vi "Utility_Calculate_PS.vi"(5 "input_2":dbl=84000.0, 7 "input_1":dbl=6.772222028271756, 8 "error in":errorcluster, 9 "units":enum16{"SI", "IP"}(ring), 10 "InpCode":T3(ring)=enum."PS", 11 "Mixure Cluster":T1={"Mixture Name"="Air (dry)", "Molecular weight (g/mol)"=28.958600656, "Critical temperature (K)"=132.83069752889762, "Critical Pressure (kPa)"=3852.042257237323, "Critical Density (mol/L)"=0.0, "# Components"=3, "Fluid File Paths"=[path "C:/Users/ASITest/Desktop/REFPROP/fluids/NITROGEN.FLD", path "C:/Users/ASITest/Desktop/REFPROP/fluids/ARGON.FLD", path "C:/Users/ASITest/Desktop/REFPROP/fluids/OXYGEN.FLD"], "Component molar fractions"=[0.7812, 0.0092, 0.2096], "Refprop Main Directory"=path "C:/Users/ASITest/Desktop/REFPROP", "DLL Version Number"=10.0}) -> (0 "error out":errorcluster={"status"=TRUE, "code"=17, "source"="REFPROP_ErrorConverter.vi<ERR>\nOne or more inputs are out of range; Temperature above 1.5x(upper limit): T = 10181.4 K, Tmax = 1993.69 K.                                                                                                                                                    \n\n\n<b>Complete call chain:</b>\r\n     REFPROP_ErrorConverter.vi\r\n     PSFLSHdll.vi\r\n     Utility_Calculate_PS.vi"}, 2 "INFO_OUT":T2={"icomp out"=3, "wmm out"=0.0, "ttrp out"=0.0, "tnbpt out"=0.0, "tc out"=0.0, "pc out"=0.0, "dc out"=0.0, "Zc out"=0.0, "acf out"=0.0, "dip out"=0.0, "Rgas out"=0.0}, 3 "dataout":dbl[](array[numeric])=[9908.201736464158, 6.772222028271756, 13169.831204666785, 84000.0, 0.0023166880524800003, 0.0023166880524800003, 10246.596882712158, 1.0691855582717507, 1.3563012835972652, 1925.6787564705157, 998.0])   [LabVIEW 2016]
doc: "Utility function that provides access to all of the functionality contained in the FLSH and SAT polymorphic VIs. \n\nPlease feel free to contact me if you have any questions .\nMy mail:ken_pop@tom.com yan.ding@jci.com"
uses:
  Ctl/Mixture Composition cluster_d.ctl
  Ctl/variable_refprop.ctl
  Ctl/FLSH_Inputs.ctl
  VIs/PSFLSHdll.vi
  VIs/HSFLSHdll.vi
  VIs/SATTdll.vi
  VIs/SATPdll.vi
  VIs/TPFLSHdll.vi
  VIs/THFLSHdll.vi
  VIs/TSFLSHdll.vi
  VIs/PHFLSHdll.vi
  VIs/PQFLSHdll.vi
  VIs/TQFLSHdll.vi
panel:
  out "n":i32=3
  out "wm":dbl=28.958600656
  out "x":dbl[](array[numeric])=[0.7812, 0.0092, 0.2096]
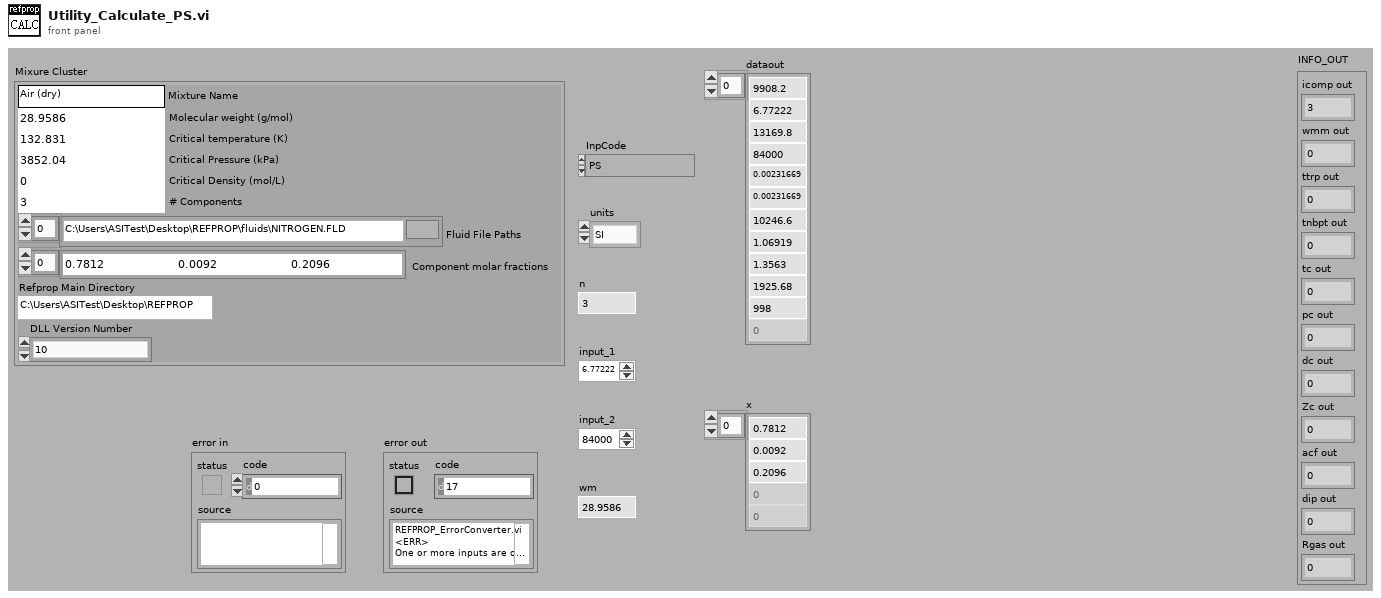
[diagram p1: front panel]
types:
  T1 = typedef "Mixture Composition cluster_d.ctl" = cluster{"Mixture Name":string, "Molecular weight (g/mol)":dbl, "Critical temperature (K)":dbl, "Critical Pressure (kPa)":dbl, "Critical Density (mol/L)":dbl, "# Components":i32, "Fluid File Paths":path[], "Component molar fractions":dbl[], "Refprop Main Directory":path, "DLL Version Number":dbl}
  T2 = cluster{"icomp out":i32, "wmm out":dbl, "ttrp out":dbl, "tnbpt out":dbl, "tc out":dbl, "pc out":dbl, "dc out":dbl, "Zc out":dbl, "acf out":dbl, "dip out":dbl, "Rgas out":dbl}
  T3 = enum16{"0", "PS", "HS", "T", "P", "TP", "TH", "TS", "PH", "PQ", "TQ"}
  T4 = typedef "FLSH_Inputs.ctl" = cluster{"t":dbl, "p":dbl, "e":dbl, "h":dbl, "s":dbl, "q":dbl, "z":dbl[], "kq":i32, "kr":i32, "D":dbl}
  T5 = typedef "variable_refprop.ctl" = cluster{"t":dbl, "p":dbl, "z":dbl[], "d":dbl, "D":dbl, "Dl":dbl, "Dv":dbl, "x":dbl[], "y":dbl[], "q":dbl, "e":dbl, "h":dbl, "s":dbl, "Cv":dbl, "Cp":dbl, "w":dbl, "ierr":i32, "herr":string, "i":i32, "z":dbl, "kq":i32, "kph":i32, "kr":i32, "nroot":i32, "k1":i32, "t1":dbl, "p1":dbl, "d1":dbl, "k2":i32, "t2":dbl, "p2":dbl, "d2":dbl, "k3":i32, "t3":dbl, "p3":dbl, "d3":dbl, "iGuess":dbl}
  T6 = typedef "FLSH_Outputs.ctl" = cluster{"t":dbl, "p":dbl, "D":dbl, "Dl":dbl, "Dv":dbl, "x":dbl[], "y":dbl[], "q":dbl, "e":dbl, "h":dbl, "s":dbl, "Cv":dbl, "Cp":dbl, "w":dbl, "ierr":i32, "herr":string, "herr_Length":i32}
  T7 = typedef "SAT_Outputs.ctl" = cluster{"D":dbl, "e":dbl, "h":dbl, "p":dbl, "s":dbl, "t":dbl, "q":dbl, "Dl":dbl, "Dv":dbl, "x":dbl[], "y":dbl[], "nroot":i32, "k1":i32, "t1":dbl, "p1":dbl, "d1":dbl, "k2":i32, "t2":dbl, "p2":dbl, "d2":dbl, "k3":i32, "t3":dbl, "p3":dbl, "d3":dbl, "ierr":i32, "herr":string, "herr_length":i32}
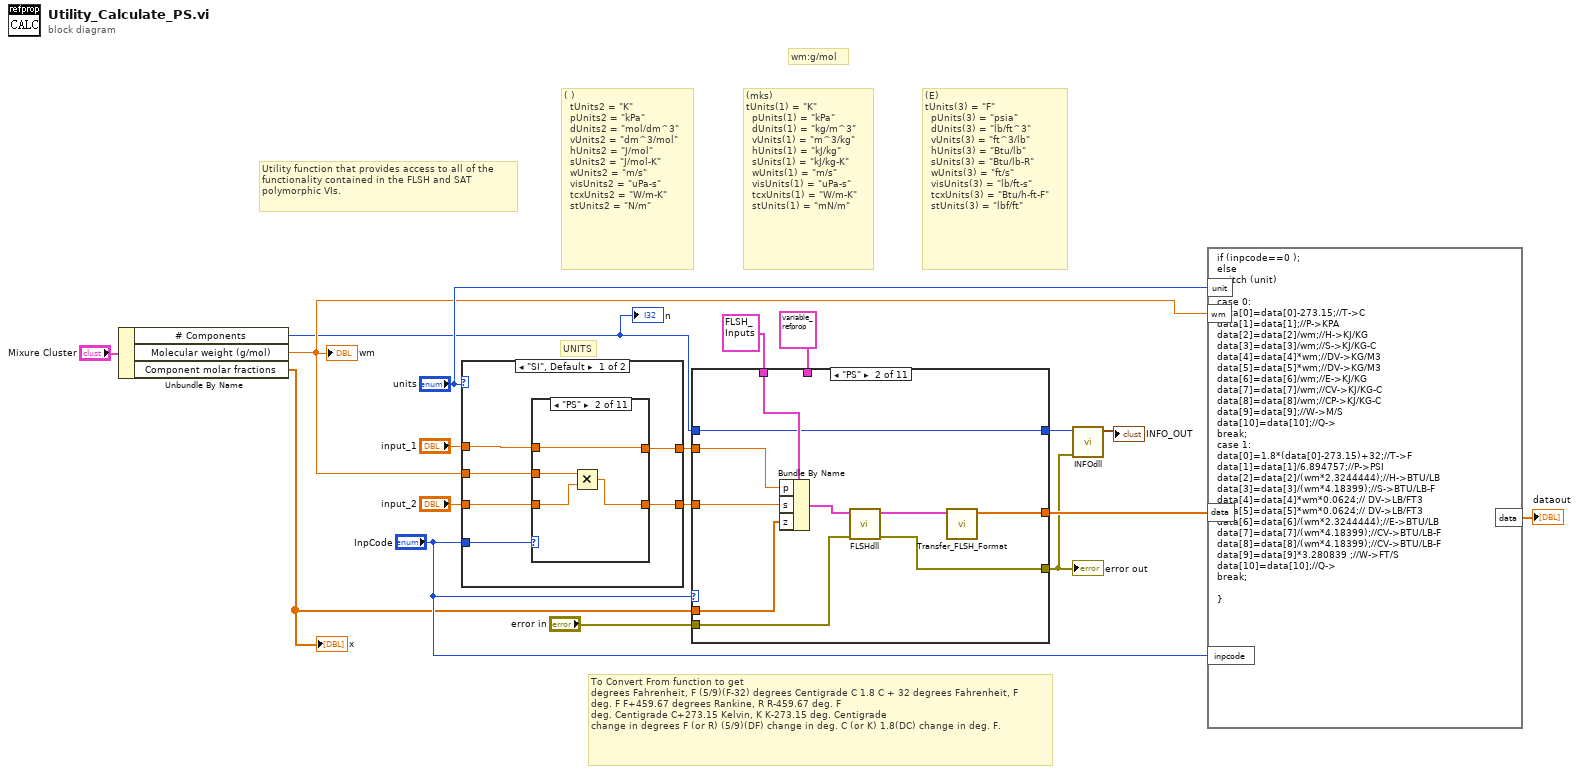
[diagram p0: block diagram]
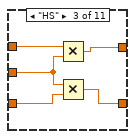
[diagram p3: hidden frame]
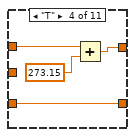
[diagram p4: hidden frame]
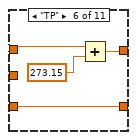
[diagram p6: hidden frame]
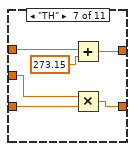
[diagram p7: hidden frame]
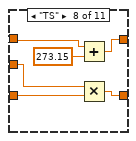
[diagram p8: hidden frame]
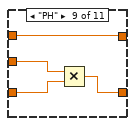
[diagram p9: hidden frame]
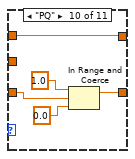
[diagram p10: hidden frame]
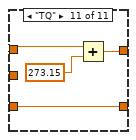
[diagram p11: hidden frame]
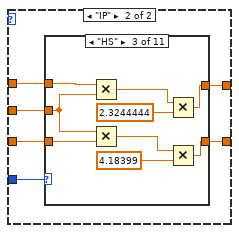
[diagram p12: hidden frame]
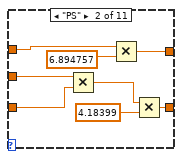
[diagram p14: hidden frame]
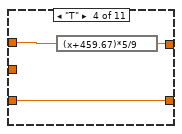
[diagram p15: hidden frame]
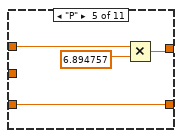
[diagram p16: hidden frame]
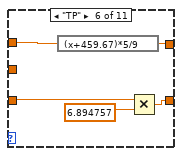
[diagram p17: hidden frame]
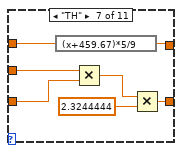
[diagram p18: hidden frame]
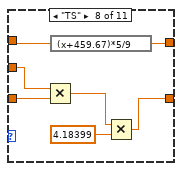
[diagram p19: hidden frame]
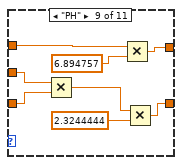
[diagram p20: hidden frame]
diagram:
  # "Utility function that provides access to all of the functionality contained in the FLSH and SAT polymorphic VIs."
  # "To Convert From function to get \ndegrees Fahrenheit, F (5/9)(F-32) degrees Centigrade C 1.8 C + 32 degrees Fahrenheit, F \ndeg. F F+459.67 degrees Rankine, R R-459.67 deg. F \ndeg. Centigrade C+273.15 Kelvin, K K-273.15 deg. Centigrade \nchange in degrees F (or R) (5/9)(DF) change in deg. C (or K) 1.8(DC) change in deg. F."
  # "(E)\ntUnits(3) = \"F\"\n  pUnits(3) = \"psia\"\n  dUnits(3) = \"lb/ft^3\"\n  vUnits(3) = \"ft^3/lb\"\n  hUnits(3) = \"Btu/lb\"\n  sUnits(3) = \"Btu/lb-R\"\n  wUnits(3) = \"ft/s\"\n  visUnits(3) = \"lb/ft-s\"\n  tcxUnits(3) = \"Btu/h-ft-F\"\n  stUnits(3) = \"lbf/ft\""
  # "(mks)\ntUnits(1) = \"K\"\n  pUnits(1) = \"kPa\"\n  dUnits(1) = \"kg/m^3\"\n  vUnits(1) = \"m^3/kg\"\n  hUnits(1) = \"kJ/kg\"\n  sUnits(1) = \"kJ/kg-K\"\n  wUnits(1) = \"m/s\"\n  visUnits(1) = \"uPa-s\"\n  tcxUnits(1) = \"W/m-K\"\n  stUnits(1) = \"mN/m\""
  # "( )\n  tUnits2 = \"K\"\n  pUnits2 = \"kPa\"\n  dUnits2 = \"mol/dm^3\"\n  vUnits2 = \"dm^3/mol\"\n  hUnits2 = \"J/mol\"\n  sUnits2 = \"J/mol-K\"\n  wUnits2 = \"m/s\"\n  visUnits2 = \"uPa-s\"\n  tcxUnits2 = \"W/m-K\"\n  stUnits2 = \"N/m\""
  # "wm:g/mol"
  # "UNITS"
  n1 = Unbundle By Name("Mixure Cluster") -> ("# Components"=w2:i32, "Molecular weight (g/mol)"=w6:dbl, "Component molar fractions"=w5:dbl[])
  "x" <- w5
  "wm" <- w6
  "n" <- w2
  n2 = case shown="\"SI\", Default" "units" {
    tunnel: "InpCode" -> [w24 w71]
    tunnel: "input_1" -> [w23 w74]
    tunnel: [w22 w76] -> w16
    tunnel: "input_2" -> [w21 w72]
    tunnel: [w20 w75] -> w14
    tunnel: w6 -> [w19 w73]
    frame "SI", Default {
      n3 = case shown="\"PS\"" w24 {
        tunnel: w23 -> [w26 w30 w35 w38 w41 w44 w50 w56 w58 w64 w69]
        tunnel: [w26 w30 w31 w37 w41 w43 w49 w55 w58 w64 w68] -> w22
        tunnel: w21 -> [w25 w28 w33 w36 w40 w42 w47 w53 w60 w63 w67]
        tunnel: [w25 w27 w32 w36 w40 w42 w46 w52 w59 w62 w67] -> w20
        tunnel: w19 -> [_ w29 w34 _ _ _ w48 w54 w61 _ _]
        frame "0", Default {
        }
        frame "PS" {
          n4 = Multiply(x=w29, y=w28) -> (x*y=w27:dbl)
        }
        frame "HS" {
          n5 = Multiply(x=w35, y=w34) -> (x*y=w31:dbl)
          n6 = Multiply(x=w34, y=w33) -> (x*y=w32:dbl)
        }
        frame "T" {
          n7 = Add(x=w38, y=273.15) -> (x+y=w37:dbl)
        }
        frame "P" {
        }
        frame "TP" {
          n8 = Add(x=w44, y=273.15) -> (x+y=w43:dbl)
        }
        frame "TH" {
          n9 = Add(x=w50, y=273.15) -> (x+y=w49:dbl)
          n10 = Multiply(x=w48, y=w47) -> (x*y=w46:dbl)
        }
        frame "TS" {
          n11 = Add(x=w56, y=273.15) -> (x+y=w55:dbl)
          n12 = Multiply(x=w54, y=w53) -> (x*y=w52:dbl)
        }
        frame "PH" {
          n13 = Multiply(x=w61, y=w60) -> (x*y=w59:dbl)
        }
        frame "PQ" {
          n14 = In Range and Coerce(upper limit=1.0 ("上限"), x=w63, lower limit=0.0 ("下限")) -> (coerced(x)=w62:dbl)  [unwired: 1 out]
        }
        frame "TQ" {
          n15 = Add(x=w69, y=273.15) -> (x+y=w68:dbl)
        }
      }
    }
    frame "IP" {
      n16 = case shown="\"HS\"" w71 {
        tunnel: w74 -> [w78 w83 w95 w97 w100 w104 w109 w116 w126 w131 w139]
        tunnel: [w78 w82 w87 w96 w99 w103 w108 w115 w125 w130 w138] -> w76
        tunnel: w72 -> [w77 w85 w93 w98 w102 w106 w113 w120 w128 w134 w137]
        tunnel: [w77 w79 w90 w98 w102 w105 w110 w117 w122 w133 w137] -> w75
        tunnel: w73 -> [_ w86 w94 _ _ _ w114 w121 w129 _ _]
        frame "0", Default {
        }
        frame "PS" {
          n17 = Multiply(x=w86, y=w85) -> (x*y=w80:dbl)
          n18 = Multiply(x=w83, y=6.894757) -> (x*y=w82:dbl)
          n19 = Multiply(x=w80, y=4.18399) -> (x*y=w79:dbl)
        }
        frame "HS" {
          n20 = Multiply(x=w95, y=w94) -> (x*y=w88:dbl)
          n21 = Multiply(x=w94, y=w93) -> (x*y=w91:dbl)
          n22 = Multiply(x=w88, y=2.3244444) -> (x*y=w87:dbl)
          n23 = Multiply(x=w91, y=4.18399) -> (x*y=w90:dbl)
        }
        frame "T" {
          n24 = expression code="(x+459.67)*5/9"(w97) -> (w96:dbl)
        }
        frame "P" {
          n25 = Multiply(x=w100, y=6.894757) -> (x*y=w99:dbl)
        }
        frame "TP" {
          n26 = expression code="(x+459.67)*5/9"(w104) -> (w103:dbl)
          n27 = Multiply(x=w106, y=6.894757) -> (x*y=w105:dbl)
        }
        frame "TH" {
          n28 = expression code="(x+459.67)*5/9"(w109) -> (w108:dbl)
          n29 = Multiply(x=w114, y=w113) -> (x*y=w111:dbl)
          n30 = Multiply(x=w111, y=2.3244444) -> (x*y=w110:dbl)
        }
        frame "TS" {
          n31 = Multiply(x=w121, y=w120) -> (x*y=w118:dbl)
          n32 = expression code="(x+459.67)*5/9"(w116) -> (w115:dbl)
          n33 = Multiply(x=w118, y=4.18399) -> (x*y=w117:dbl)
        }
        frame "PH" {
          n34 = Multiply(x=w129, y=w128) -> (x*y=w123:dbl)
          n35 = Multiply(x=w126, y=6.894757) -> (x*y=w125:dbl)
          n36 = Multiply(x=w123, y=2.3244444) -> (x*y=w122:dbl)
        }
        frame "PQ" {
          n37 = In Range and Coerce(upper limit=1.0 ("上限"), x=w134, lower limit=0.0 ("下限")) -> (coerced(x)=w133:dbl)  [unwired: 1 out]
          n38 = Multiply(x=w131, y=6.894757) -> (x*y=w130:dbl)
        }
        frame "TQ" {
          n39 = expression code="(x+459.67)*5/9"(w139) -> (w138:dbl)
        }
      }
    }
  }
  n40 = case shown="\"PS\"" "InpCode" {
    tunnel: w5 -> [_ w148 w158 w170 w178 w186 w199 w207 w220 w229 w239]
    tunnel: "error in" -> [w144 w154 w163 w173 w181 w192 w201 w212 w222 w231 w241]
    tunnel: [w144 w153 w162 w172 w182 w188 w200 w211 w221 w230 w240] -> w1
    tunnel: w16 -> [_ w151 w160 w171 w179 w190 w198 w209 w219 w228 w237]
    tunnel: w14 -> [_ w150 w161 _ _ w191 w197 w210 w218 w227 w238]
    tunnel: w2 -> [w140 w147 w157 w165 w174 w183 w195 w205 w215 w225 w235]
    tunnel: [w141 w146 w155 w166 w175 w185 w193 w204 w213 w223 w234] -> w13
    tunnel: T5 {"t"=0.0, "p"=0.0, "z"=[0.0, 0.0, 0.0, 0.0, 0.0, 0.0, 0.0, 0.0, 0.0, 0.0, 0.0, 0.0, 0.0, 0.0, 0.0, 0.0, 0.0, 0.0, 0.0, 0.0], "d"=0.0, "D"=0.0, "Dl"=0.0, "Dv"=0.0, "x"=[0.0, 0.0, 0.0, 0.0, 0.0, 0.0, 0.0, 0.0, 0.0, 0.0, 0.0, 0.0, 0.0, 0.0, 0.0, 0.0, 0.0, 0.0, 0.0, 0.0], "y"=[0.0, 0.0, 0.0, 0.0, 0.0, 0.0, 0.0, 0.0, 0.0, 0.0, 0.0, 0.0, 0.0, 0.0, 0.0, 0.0, 0.0, 0.0, 0.0, 0.0], "q"=0.0, "e"=0.0, "h"=0.0, "s"=0.0, "Cv"=0.0, "Cp"=0.0, "w"=0.0, "ierr"=0, "herr"="", "i"=0, "z"=0.0, "kq"=0, "kph"=0, "kr"=0, "nroot"=0, "k1"=0, "t1"=0.0, "p1"=0.0, "d1"=0.0, "k2"=0, "t2"=0.0, "p2"=0.0, "d2"=0.0, "k3"=0, "t3"=0.0, "p3"=0.0, "d3"=0.0, "iGuess"=0.0} ("variable") -> [_ _ _ _ _ _ _ _ _ _ _]
    tunnel: [w140 w147 w157 w165 w174 w183 w195 w205 w215 w225 w235] -> w3
    tunnel: T4 {"t"=0.0, "p"=0.0, "e"=0.0, "h"=0.0, "s"=0.0, "q"=0.0, "z"=[0.0, 0.0, 0.0, 0.0, 0.0, 0.0, 0.0, 0.0, 0.0, 0.0, 0.0, 0.0, 0.0, 0.0, 0.0, 0.0, 0.0, 0.0, 0.0, 0.0], "kq"=0, "kr"=0, "D"=0.0} ("FLSH Inputs") -> [_ w149 w159 _ _ w187 w196 w208 w217 w226 w236]
    frame "0", Default {
      n41 = Initialize Array(0.0 ("元素"), 10 ("维数大小")) -> (w141:dbl[])
    }
    frame "PS" {
      n42 = Bundle By Name(cluster=w149, "p"=w151, "s"=w150, "z"=w148) -> (w152:T4)
      n43 = call-poly "FLSHdll.vi"("error in (no error)"=w154, "FLSH Inputs"=w152) -> ("error out"=w153:errorcluster, "FLSH Outputs"=w145:T6)  [unwired: 8 in]
      n44 = call "Transfer_FLSH_Format.vi"("FLSH Outputs"=w145) -> ("Array out"=w146:dbl[])  [unwired: 10 in]
    }
    frame "HS" {
      n45 = Bundle By Name(cluster=w159, "h"=w160, "s"=w161, "z"=w158) -> (w164:T4)
      n46 = call-poly "FLSHdll.vi"("error in (no error)"=w163, "FLSH Inputs"=w164) -> ("error out"=w162:errorcluster, "FLSH Outputs"=w156:T6)  [unwired: 8 in]
      n47 = call "Transfer_FLSH_Format.vi"("FLSH Outputs"=w156) -> ("Array out"=w155:dbl[])  [unwired: 10 in]
    }
    frame "T" {
      n48 = Bundle By Name(cluster=cluster{"t":dbl, "z":dbl[], "kph":u16} {"t"=0.0, "z"=[0.0, 0.0, 0.0, 0.0, 0.0, 0.0, 0.0, 0.0, 0.0, 0.0, 0.0, 0.0, 0.0, 0.0, 0.0, 0.0, 0.0, 0.0, 0.0, 0.0], "kph"=2} ("SAT Inputs"), "t"=w171, "z"=w170, "kph"=w165) -> (w169:cluster{"t":dbl, "z":dbl[], "kph":u16})
      n49 = call-poly "SAT.vi"("error in (no error)"=w173, "SAT Inputs"=w169) -> ("error out"=w172:errorcluster, "SAT Outputs"=w167:T7)  [unwired: 8 in]
      n50 = call "Transfer_SAT_Format.vi"("SAT Outputs"=w167) -> ("Array out"=w166:dbl[])  [unwired: 10 in]
    }
    frame "P" {
      n51 = Bundle By Name(cluster=cluster{"p":dbl, "z":dbl[], "kph":u16} {"p"=0.0, "z"=[0.0, 0.0, 0.0, 0.0, 0.0, 0.0, 0.0, 0.0, 0.0, 0.0, 0.0, 0.0, 0.0, 0.0, 0.0, 0.0, 0.0, 0.0, 0.0, 0.0], "kph"=4} ("SAT Inputs"), "p"=w179, "z"=w178, "kph"=w174) -> (w177:cluster{"p":dbl, "z":dbl[], "kph":u16})
      n52 = call-poly "SAT.vi"("error in (no error)"=w181, "SAT Inputs"=w177) -> ("error out"=w182:errorcluster, "SAT Outputs"=w176:T7)  [unwired: 8 in]
      n53 = call "Transfer_SAT_Format.vi"("SAT Outputs"=w176) -> ("Array out"=w175:dbl[])  [unwired: 10 in]
    }
    frame "TP" {
      n54 = Bundle By Name(cluster=w187, "t"=w190, "p"=w191, "z"=w186) -> (w189:T4)
      n55 = call-poly "FLSHdll.vi"("error in (no error)"=w192, "FLSH Inputs"=w189) -> ("error out"=w188:errorcluster, "FLSH Outputs"=w184:T6)  [unwired: 8 in]
      n56 = call "Transfer_FLSH_Format.vi"("FLSH Outputs"=w184) -> ("Array out"=w185:dbl[])  [unwired: 10 in]
    }
    frame "TH" {
      n57 = Bundle By Name(cluster=w196, "t"=w198, "h"=w197, "kr"=w195, "z"=w199) -> (w202:T4)
      n58 = call-poly "FLSHdll.vi"("error in (no error)"=w201, "FLSH Inputs"=w202) -> ("error out"=w200:errorcluster, "FLSH Outputs"=w194:T6)  [unwired: 8 in]
      n59 = call "Transfer_FLSH_Format.vi"("FLSH Outputs"=w194) -> ("Array out"=w193:dbl[])  [unwired: 10 in]
    }
    frame "TS" {
      n60 = Bundle By Name(cluster=w208, "t"=w209, "s"=w210, "kr"=w205, "z"=w207) -> (w206:T4)
      n61 = call-poly "FLSHdll.vi"("error in (no error)"=w212, "FLSH Inputs"=w206) -> ("error out"=w211:errorcluster, "FLSH Outputs"=w203:T6)  [unwired: 8 in]
      n62 = call "Transfer_FLSH_Format.vi"("FLSH Outputs"=w203) -> ("Array out"=w204:dbl[])  [unwired: 10 in]
    }
    frame "PH" {
      n63 = Bundle By Name(cluster=w217, "p"=w219, "h"=w218, "z"=w220) -> (w216:T4)
      n64 = call-poly "FLSHdll.vi"("error in (no error)"=w222, "FLSH Inputs"=w216) -> ("error out"=w221:errorcluster, "FLSH Outputs"=w214:T6)  [unwired: 8 in]
      n65 = call "Transfer_FLSH_Format.vi"("FLSH Outputs"=w214) -> ("Array out"=w213:dbl[])  [unwired: 10 in]
    }
    frame "PQ" {
      n66 = Bundle By Name(cluster=w226, "p"=w228, "q"=w227, "kq"=w225, "z"=w229) -> (w232:T4)
      n67 = call-poly "FLSHdll.vi"("error in (no error)"=w231, "FLSH Inputs"=w232) -> ("error out"=w230:errorcluster, "FLSH Outputs"=w224:T6)  [unwired: 8 in]
      n68 = call "Transfer_FLSH_Format.vi"("FLSH Outputs"=w224) -> ("Array out"=w223:dbl[])  [unwired: 10 in]
    }
    frame "TQ" {
      n69 = Bundle By Name(cluster=w236, "t"=w237, "q"=w238, "kq"=w235, "z"=w239) -> (w242:T4)
      n70 = call-poly "FLSHdll.vi"("error in (no error)"=w241, "FLSH Inputs"=w242) -> ("error out"=w240:errorcluster, "FLSH Outputs"=w233:T6)  [unwired: 8 in]
      n71 = call "Transfer_FLSH_Format.vi"("FLSH Outputs"=w233) -> ("Array out"=w234:dbl[])  [unwired: 10 in]
    }
  }
  "error out" <- w1
  n72 = call "INFOdll.vi"("error in (no error)"=w1, "icomp"=w3) -> ("INFO_OUT"=→"INFO_OUT":T2)  [unwired: 8 in, 1 out]
  n73 = formula code="if (inpcode==0 );\nelse\nswitch (unit)\n{\ncase 0:\ndata[0]=data[0]-273.15;//T->C\ndata[1]=data[1];//P->KPA\ndata[2]=data[2]/wm;//H->KJ/KG\ndata[3]=data[3]/wm;//S->KJ/KG-C\ndata[4]=data[4]*wm;//DV->KG/M3\ndata[5]=data[5]*wm;//DV->KG/M3\ndata[6]=data[6]/wm;//E->KJ/KG\ndata[7]=data[7]/wm;//CV->KJ/KG-C\ndata[8]=data[8]/wm;//CP->KJ/KG-C\ndata[9]=data[9];//W->M/S\ndata[10]=data[10];//Q->\nbreak;\ncase 1:\ndata[0]=1.8*(data[0]-273.15)+32;//T->F\ndata[1]=data[1]/6.894757;//P->PSI\ndata[2]=data[2]/(wm*2.3244444);//H->BTU/LB\ndata[3]=data[3]/(wm*4.18399);//S->BTU/LB-F\ndata[4]=data[4]*wm*0.0624;// DV->LB/FT3\ndata[5]=data[5]*wm*0.0624;// DV->LB/FT3\ndata[6]=data[6]/(wm*2.3244444);//E->BTU/LB\ndata[7]=data[7]/(wm*4.18399);//CV->BTU/LB-F\ndata[8]=data[8]/(wm*4.18399);//CV->BTU/LB-F\ndata[9]=data[9]*3.280839 ;//W->FT/S\ndata[10]=data[10];//Q->\nbreak;\n\n}"("data"=w13, "unit"="units", "inpcode"="InpCode", "wm"=w6) -> ("data"=→"dataout":dbl[])
